vi "binary_reader Old.vi"(7 "error in":errorcluster, 10 "path to binary file":path) -> (0 "error out":errorcluster)   [LabVIEW 2019]
uses:
  Controls/gyro_control_memory_structure.ctl
  Controls/gyro_control_measurement_settings.ctl
  Controls/gyro_control_time_informations.ctl
  Controls/gyro_control_measurement_data.ctl
  Controls/gyro_control_all_in_one_package.ctl
panel:
  out "Misc":T3 {"time informations"."length" format="%<%H:%M:%S%3u>t"; "actigraph settings"."id" format="%02d"; "actigraph settings"."xlRange" format="%02x"; "actigraph settings"."ODR" format="%02x"}
  out "3 axis acceleration in time":waveform(dbl)[](graph)
  out "voltage over time":waveform(dbl)(graph)
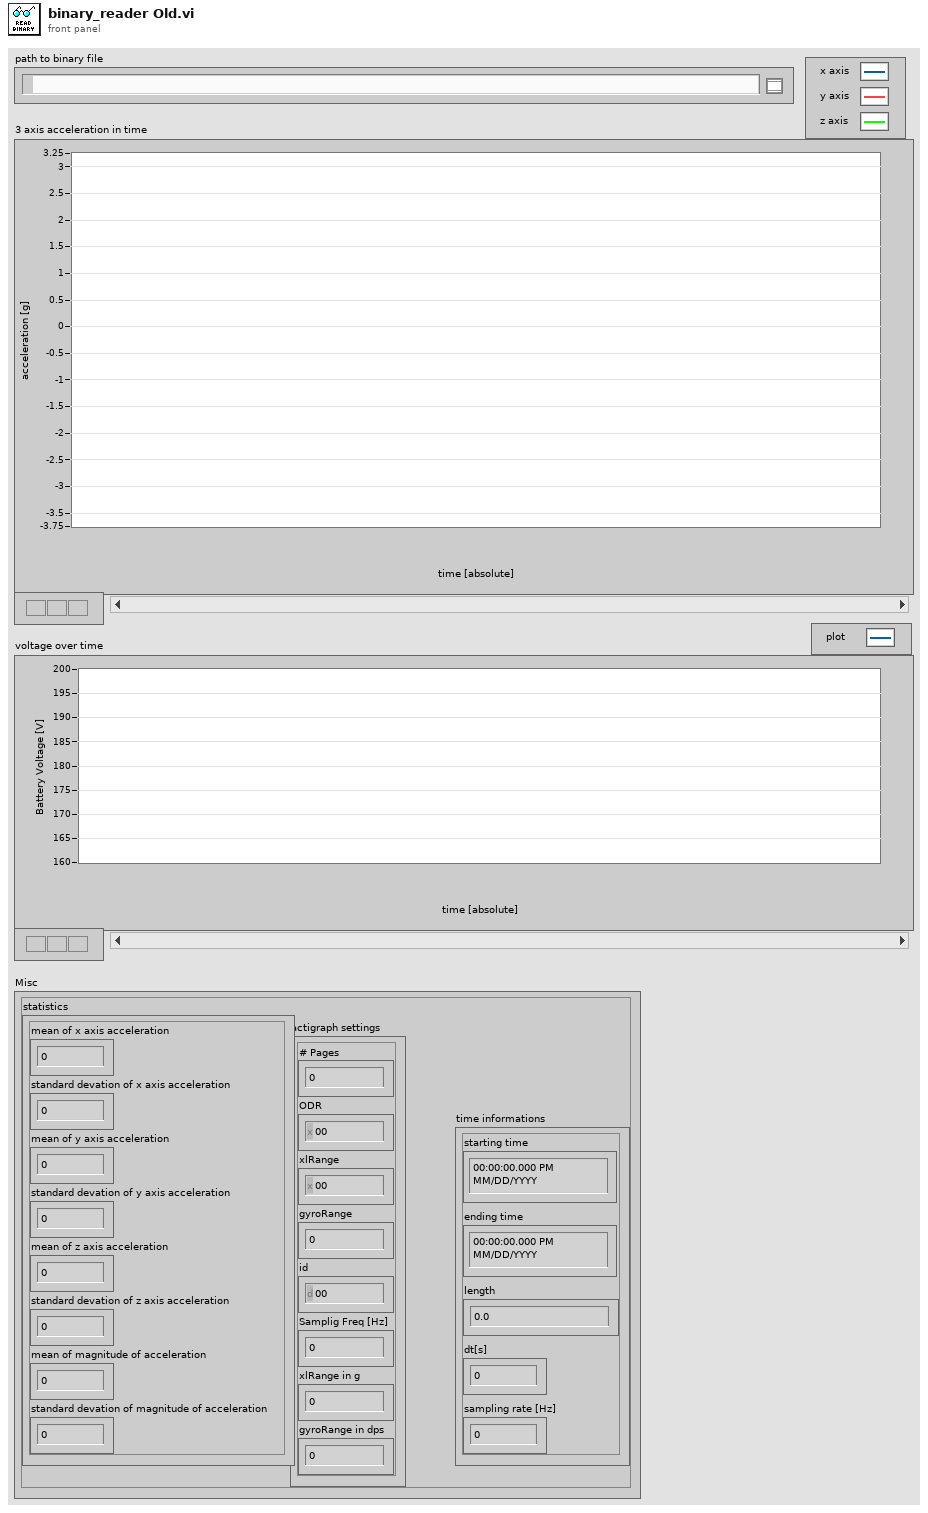
[diagram p1: front panel]
types:
  T1 = typedef "gyro_control_time_informations.ctl" = cluster{"starting time":timestamp, "ending time":timestamp, "dt[s]":dbl, "sampling rate [Hz]":dbl, "length":dbl}
  T2 = typedef "gyro_control_measurement_settings.ctl" = cluster{"# Pages":i32, "ODR":u8, "xlRange":u8, "gyroRange":u8, "id":u8, "Samplig Freq [Hz]":dbl, "xlRange in g":dbl, "gyroRange in dps":dbl}
  T3 = cluster{"statistics":cluster{"mean of x axis acceleration":dbl, "standard devation of x axis acceleration":dbl, "mean of y axis acceleration":dbl, "standard devation of y axis acceleration":dbl, "mean of z axis acceleration":dbl, "standard devation of z axis acceleration":dbl, "mean of magnitude of acceleration":dbl, "standard devation of magnitude of acceleration":dbl}, "time informations":T1, "actigraph settings":T2}
  T4 = typedef "gyro_control_memory_structure.ctl" = cluster{"length of metadata [byte]":i32, "length of page [byte]":i32, "length of measurement \ndata on page [byte]":i32, "length of dataset [byte]":i32}
  T5 = typedef "gyro_control_all_in_one_package.ctl" = cluster{"measurement data":T6, "actigraph settings":T2, "memory structure":T4, "time informations":T1}
  T6 = typedef "gyro_control_measurement_data.ctl" = cluster{"number of samples per axis":i32, "timestamp array":dbl[], "offset array":dbl[], "x, y, z axis data":waveform(dbl)[], "magnitude of acceleartion vectors":waveform(dbl), "statistics":cluster{"mean of x axis acceleration":dbl, "standard devation \nof x axis acceleration":dbl, "mean of y axis acceleration":dbl, "standard devation \nof y axis acceleration":dbl, "mean of z axis acceleration":dbl, "standard devation \nof z axis acceleration":dbl, "mean of magnitude\n of acceleration":dbl, "standard devation \nof magnitude of acceleration":dbl}, "voltage":waveform(dbl)}
  T7 = typedef "control_all_in_one_package.ctl" = cluster{"memory structure":T8, "actigraph settings":T9, "time informations":T10, "measurement data":T11}
  T8 = typedef "control_memory_structure.ctl" = cluster{"length of metadata [byte]":i32, "length of page [byte]":i32, "length of measurement data on page [byte]":i32, "length of dataset [byte]":i32}
  T9 = typedef "control_measurement_settings.ctl" = cluster{"sampling frequency [Hz]":dbl, "measurement interval [± g]":i32, "high precision?":bool, "number of pages":i32, "rate code":i32, "range code":i32, "id":i32}
  T10 = typedef "control_time_informations.ctl" = cluster{"starting time":timestamp, "ending time":timestamp, "dt[s]":dbl, "sampling rate [Hz]":dbl, "length":dbl}
  T11 = typedef "control_measurement_data.ctl" = cluster{"number of samples per axis":i32, "timestamp array":dbl[], "offset array":dbl[], "x, y, z axis data":waveform(dbl)[], "normalised magnitude of acceleartion vectors":waveform(dbl), "calibration coefficients":T12, "statistics":T13, "battery voltage":waveform(dbl), "magnitude of acceleartion vectors":waveform(dbl)}
  T12 = typedef "control_calibration_coefficients.ctl" = cluster{"Sx":dbl, "Ox":dbl, "Sy":dbl, "Oy":dbl, "Sz":dbl, "Oz":dbl}
  T13 = typedef "control_statistics.ctl" = cluster{"mean of x axis acceleration":dbl, "standard devation of x axis acceleration":dbl, "mean of y axis acceleration":dbl, "standard devation of y axis acceleration":dbl, "mean of z axis acceleration":dbl, "standard devation of z axis acceleration":dbl, "mean of normalised magnitude of acceleration":dbl, "standard devation of normalised magnitude of acceleration":dbl}
  T14 = typedef "gyro_control_all_in_one_package.ctl" = cluster{"measurement data":T6, "actigraph settings":T9, "memory structure":T4, "time informations":T1}
  T15 = cluster{"mean of x axis acceleration":dbl, "standard devation \nof x axis acceleration":dbl, "mean of y axis acceleration":dbl, "standard devation \nof y axis acceleration":dbl, "mean of z axis acceleration":dbl, "standard devation \nof z axis acceleration":dbl, "mean of magnitude\n of acceleration":dbl, "standard devation \nof magnitude of acceleration":dbl}
  T16 = cluster{"mean of x axis acceleration":dbl, "standard devation of x axis acceleration":dbl, "mean of y axis acceleration":dbl, "standard devation of y axis acceleration":dbl, "mean of z axis acceleration":dbl, "standard devation of z axis acceleration":dbl, "mean of magnitude of acceleration":dbl, "standard devation of magnitude of acceleration":dbl}
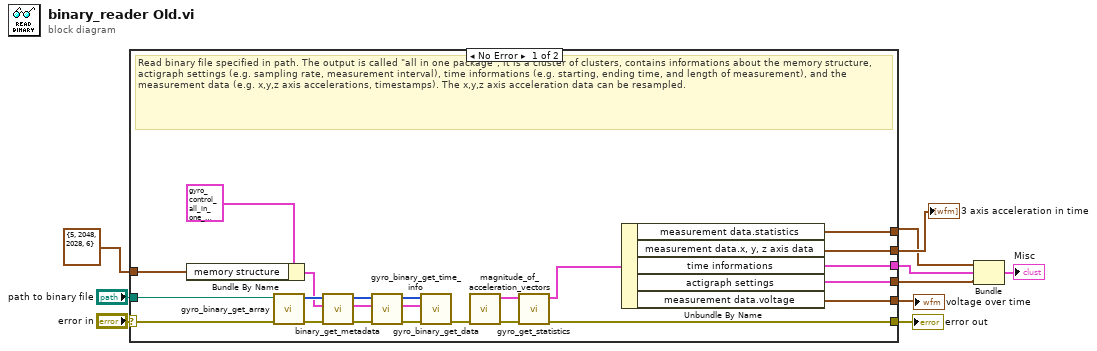
[diagram p0: block diagram]
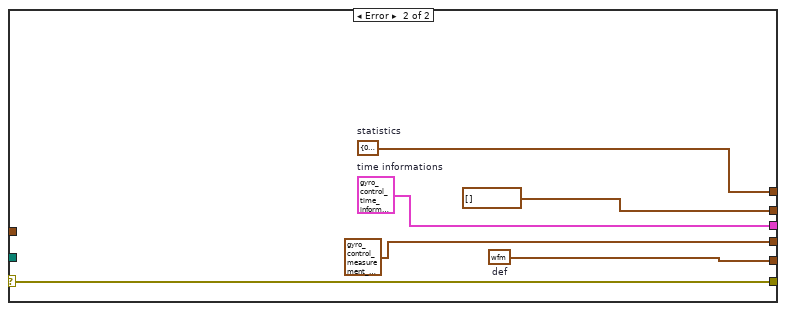
[diagram p2: hidden frame]
diagram:
  n1 = case shown="No Error" "error in" {
    selector: "error in" -> [w19 w39]
    tunnel: "path to binary file" -> [w32 _]
    tunnel: T4 {"length of metadata [byte]"=5, "length of page [byte]"=2048, "length of measurement \ndata on page [byte]"=2028, "length of dataset [byte]"=6} ("memory structure") -> [w26 _]
    tunnel: [w14 w39] -> w9
    tunnel: [w25 waveform(dbl)[] [] ("x, y, z axis data")] -> w6
    tunnel: [w22 w37] -> w3
    tunnel: [w21 T2 {"# Pages"=0, "ODR"=0, "xlRange"=0, "gyroRange"=0, "id"=0, "Samplig Freq [Hz]"=9.980607627666451, "xlRange in g"=0.0, "gyroRange in dps"=0.0} ("actigraph settings")] -> w2
    tunnel: [w15 w35] -> w4
    tunnel: [w11 w34] -> w5
    frame No Error {
      # "Read binary file specified in path. The output is called \"all in one package\", it is a cluster of clusters, contains informations about the memory structure, actigraph settings (e.g. sampling rate, measurement interval), time informations (e.g. starting, ending time, and length of measurement), and the measurement data (e.g. x,y,z axis accelerations, timestamps). The x,y,z axis acceleration data can be resampled."
      n2 = Bundle By Name(cluster=T5 {"measurement data"={"number of samples per axis"=0, "timestamp array"=[], "offset array"=[], "x, y, z axis data"=[], "magnitude of acceleartion vectors"={"t0"=timestamp(0 s since 1904-01-01), "dt"=1.0, "Y"=[]}, "statistics"={"mean of x axis acceleration"=0.0, "standard devation \nof x axis acceleration"=0.0, "mean of y axis acceleration"=0.0, "standard devation \nof y axis acceleration"=0.0, "mean of z axis acceleration"=0.0, "standard devation \nof z axis acceleration"=0.0, "mean of magnitude\n of acceleration"=0.0, "standard devation \nof magnitude of acceleration"=0.0}, "voltage"={"t0"=timestamp(0 s since 1904-01-01), "dt"=1.0, "Y"=[]}}, "actigraph settings"={"# Pages"=0, "ODR"=0, "xlRange"=0, "gyroRange"=0, "id"=0, "Samplig Freq [Hz]"=0.0, "xlRange in g"=0.0, "gyroRange in dps"=0.0}, "memory structure"={"length of metadata [byte]"=0, "length of page [byte]"=0, "length of measurement \ndata on page [byte]"=0, "length of dataset [byte]"=0}, "time informations"={"starting time"=timestamp(0 s since 1904-01-01), "ending time"=timestamp(0 s since 1904-01-01), "dt[s]"=0.0, "sampling rate [Hz]"=0.0, "length"=0.0}} ("all in one package"), "memory structure"=w26) -> (w23:T5)
      n3 = call "gyro_binary_get_array.vi"("error in"=w19, "path to binary file"=w32) -> ("error out"=w31:errorcluster, "binary data"=w29:u8[])  [unwired: 8 in]
      n4 = call "binary_get_metadata.vi"("error in"=w31, "all in one package in"=w23, "binary data w/ calibration coefficients"=w29) -> ("error out"=w33:errorcluster, "all in one package out"=w24:T7, "pages"=w30:u8[])  [unwired: 6 in]
      n5 = call "gyro_binary_get_time_info.vi"("error in"=w33, "all in one package in"=w24, "pages"=w30) -> ("error out"=w28:errorcluster, "all in one package out"=w20:T5, "pages excluding first and last page"=w27:u8[])  [unwired: 6 in]
      n6 = call "gyro_binary_get_data.vi"("error in"=w28, "all in one package in"=w20, "pages excluding first and last page"=w27) -> ("error out"=w18:errorcluster)  [unwired: 7 in, 1 out]
      n7 = call "magnitude_of_acceleration_vectors.vi"("error in"=w18) -> ("error out"=w17:errorcluster, "all in one package out"=w16:T14)  [unwired: 9 in]
      n8 = call "gyro_get_statistics.vi"("error in"=w17, "all in one package in"=w16) -> ("error out"=w14:errorcluster, "all in one package out"=w13:T14)  [unwired: 8 in]
      n9 = Unbundle By Name(w13) -> ("measurement data.statistics"=w15:T15, "measurement data.x, y, z axis data"=w25:waveform(dbl)[], "time informations"=w22:T1, "actigraph settings"=w21:T9, "measurement data.voltage"=w11:waveform(dbl))
    }
    frame Error {
      w34 = waveform(dbl) {"t0"=timestamp(0 s since 1904-01-01), "dt"=1.0, "Y"=[]}  # def
      w35 = T16 {"mean of x axis acceleration"=0.0, "standard devation of x axis acceleration"=0.0, "mean of y axis acceleration"=0.0, "standard devation of y axis acceleration"=0.0, "mean of z axis acceleration"=0.0, "standard devation of z axis acceleration"=0.0, "mean of magnitude of acceleration"=0.0, "standard devation of magnitude of acceleration"=0.0}  # statistics
      w37 = T1 {"starting time"=timestamp(0 s since 1904-01-01), "ending time"=timestamp(0 s since 1904-01-01), "dt[s]"=0.0, "sampling rate [Hz]"=0.0, "length"=0.0}  # time informations
    }
  }
  "error out" <- w9
  "3 axis acceleration in time" <- w6
  "voltage over time" <- w5
  n10 = Bundle("statistics"=w4, "time informations"=w3, "actigraph settings"=w2) -> (→"Misc":T3)  [unwired: 1 in]
